vi "Set Sensor Attributes.vi"(0 "task in":refnum<k21>, 5 "channel table":T1[](array[typedef]) {"input terminal configuration" items=["default"=-1, "RSE"=10083, "NRSE"=10078, "Differential"=10106, "Pseudodifferential"=12529]; "Channel Type" items=["Voltage (V)"=0, "Charge (C)"=9, "-"=99, "SPL (Pa)"=3, "Force (lbf)"=6, "Force (N)"=1, "Acceleration (g) - IEPE"=2, "Acceleration (g) - Charge"=12, "Acceleration (g) - 4 wire DC Voltage"=22, "Velocity (in/s)"=7, "Velocity (mm/s)"=8, "Prox Probe (mil)"=4, "Prox Probe (mm)"=5]}, 11 "error in":errorcluster) -> (4 "task out":refnum<k21>, 15 "error out":errorcluster)   [LabVIEW 2024, in "Dynamic Signal Acquisition (Interactive) UI.lvlib"]
doc: "Set SV Sensor Attributes."
uses:
  Dynamic Signal Acquisition (Interactive) UI.lvlib
  SFPDAQmx Channel Info.ctl
  <vilib>/addons/Sound and Vibration/svt_DAQmx/subVIs/sv_SetCustomAttributeDouble.vi
  <vilib>/addons/Sound and Vibration/svt_DAQmx/subVIs/sv_SetCustomAttributeString.vi
  <vilib>/addons/Sound and Vibration/svt_DAQmx/Configuration XControl/SVX NI-DAQmx AI Configuration XControl.xctl
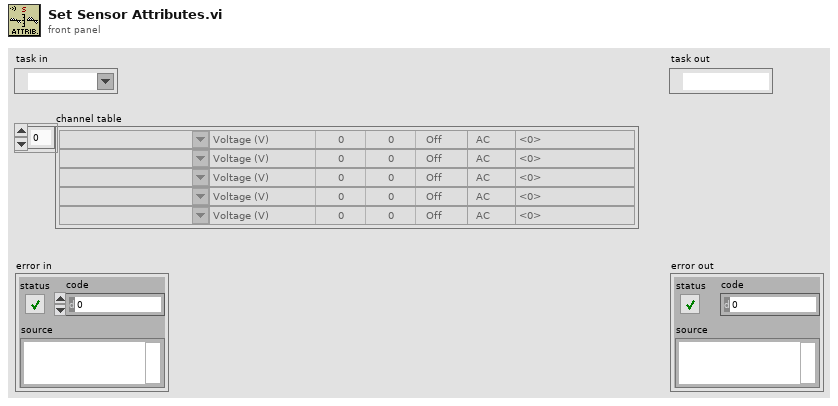
[diagram p1: front panel]
types:
  T1 = typedef "Dynamic Signal Acquisition (Interactive) UI.lvlib/SFPDAQmx Channel Info.ctl" = cluster{"Initialized?":bool, "DAQmx Channel":tag, "Channel Type":u16, "Max":dbl, "Sensitivity":dbl, "Excitation":bool, "Coupling":enum16{"AC", "DC"}, "input terminal configuration":i32, "excitation":enum16{"Off", "Min", "Max"}}
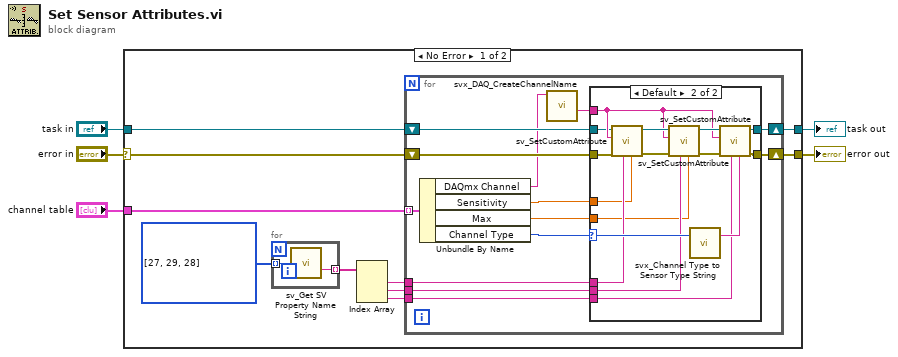
[diagram p0: block diagram]
diagram:
  n1 = case shown="No Error" "error in" {
    selector: "error in" -> [w9 w49]
    tunnel: "channel table" -> [w12 _]
    tunnel: [w11 w49] -> w4
    tunnel: [w10 w50] -> w3
    tunnel: "task in" -> [w8 w50]
    frame No Error {
      w6 = u16[] [27, 29, 28] items=["Engineering units", "Custom unit label", "Weighting filter", "Pregain", "Octave standard", "Octave bandwidth", "Octave low band", "Octave high band", "Spectrum skewed", "Samples / revolution", "Order", "Tachometer", "Pulses Per Revolution", "Rotation Direction", "Probe Angle", "Pair", "Channel Alias", "Tachometer Threshold", "Tachometer Slope", "Max Order", "Sensor Location", "Sensor Orientation", "Analog Software Trigger", "Trigger Level", "Pretrigger Samples", "Trigger Slope", "Trigger Hysteresis", "Sensor sensitivity", "Sensor type", "Sensor maximum"]
      n2 = for {
        tunnel: [w47] -> w7 mode=indexing
        tunnel: w6 -> [w48] mode=indexing
        n3 = call <vilib>:"sv_Get SV Property Name String.vi"("property"=w48) -> ("WDT attribute name"=w47:string)  [unwired: 13 in, 1 out]
      }
      n4 = Index Array(array=w7) -> (element #1=w13:string, element #2=w14:string, element #3=w15:string)  [unwired: 3 in]
      n5 = for {
        tunnel: w12 -> [w24] mode=indexing
        tunnel: w13 -> [w21]
        tunnel: w14 -> [w20]
        tunnel: w15 -> [w19]
        shift-right: [w26] -> w10
        shift-left: w8 -> [w28]
        shift-right: [w25] -> w11
        shift-left: w9 -> [w27]
        n6 = Unbundle By Name(w24) -> ("DAQmx Channel"=w23:tag, "Sensitivity"=w18:dbl, "Max"=w17:dbl, "Channel Type"=w16:u16)
        n7 = call <vilib>:"svx_DAQ_CreateChannelName.vi"("DAQmx Channel In"=w23) -> ("Channel Name"=w22:string)  [unwired: 9 in, 1 out]
        n8 = case shown="Default" w16 {
          selector: w16 -> [_ w36]
          tunnel: w22 -> [_ w41]
          tunnel: w28 -> [w30 w40]
          tunnel: [w30 w39] -> w26
          tunnel: w27 -> [w29 w38]
          tunnel: [w29 w37] -> w25
          tunnel: w21 -> [_ w35]
          tunnel: w20 -> [_ w34]
          tunnel: w19 -> [_ w33]
          tunnel: w18 -> [_ w32]
          tunnel: w17 -> [_ w31]
          frame 0, 9 {
          }
          frame Default {
            n9 = call-poly <vilib>:"sv_SetCustomAttribute.vi"("Attribute Value"=w32, "Attribute Name"=w35, "error in"=w38, "Active Channel"=w41, "task/channels in"=w40) -> ("error out"=w46:errorcluster, "task out"=w45:refnum<k21>)  [unwired: 5 in]
            n10 = call-poly <vilib>:"sv_SetCustomAttribute.vi"("Attribute Value"=w31, "Attribute Name"=w34, "error in"=w46, "Active Channel"=w41, "task/channels in"=w45) -> ("error out"=w44:errorcluster, "task out"=w43:refnum<k21>)  [unwired: 5 in]
            n11 = call <vilib>:"svx_Channel Type to Sensor Type String.vi"("channel type"=w36) -> ("sensor type"=w42:string)  [unwired: 2 in]
            n12 = call-poly <vilib>:"sv_SetCustomAttribute.vi"("Attribute Value"=w42, "Attribute Name"=w33, "error in"=w44, "Active Channel"=w41, "task/channels in"=w43) -> ("error out"=w37:errorcluster, "task out"=w39:refnum<k21>)  [unwired: 5 in]
          }
        }
      }
    }
    frame Error {
    }
  }
  "error out" <- w4
  "task out" <- w3
